vi "test_CCDGetChipTemperature.vi"(8 "error in":errorcluster) -> (0 "error out":errorcluster)   [LabVIEW 2023]
uses:
  <vilib>/addons/_JKI Toolkits/Caraya/classes/Test/Test.lvclass
  <vilib>/addons/_JKI Toolkits/Caraya/classes/Assert/Assert.lvclass
  horiba.test.lvlib
  <vilib>/addons/_JKI Toolkits/Caraya/classes/Assert/Assert Greater_Variant.vi
  <vilib>/addons/_JKI Toolkits/Caraya/classes/Assert/Assert Not Error.vi
  <vilib>/addons/_JKI Toolkits/Caraya/classes/Assert/Assert Less_Variant.vi
  Classes/CCD/CCD.lvclass
  Classes/GenericDevice/GenericDevice.lvclass
panel:
  # "Connector Pane"
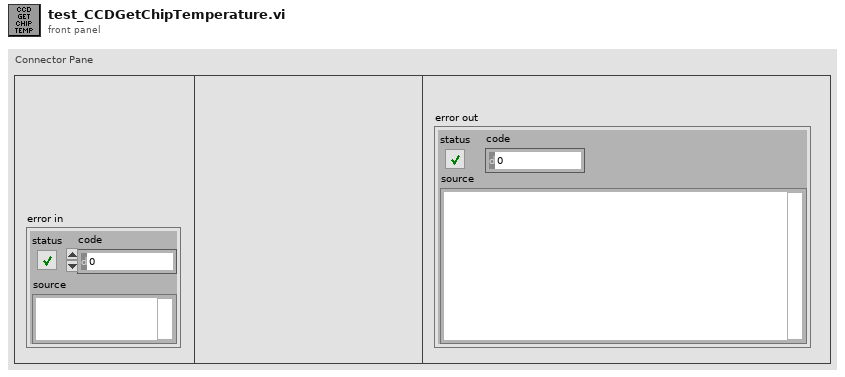
[diagram p1: front panel]
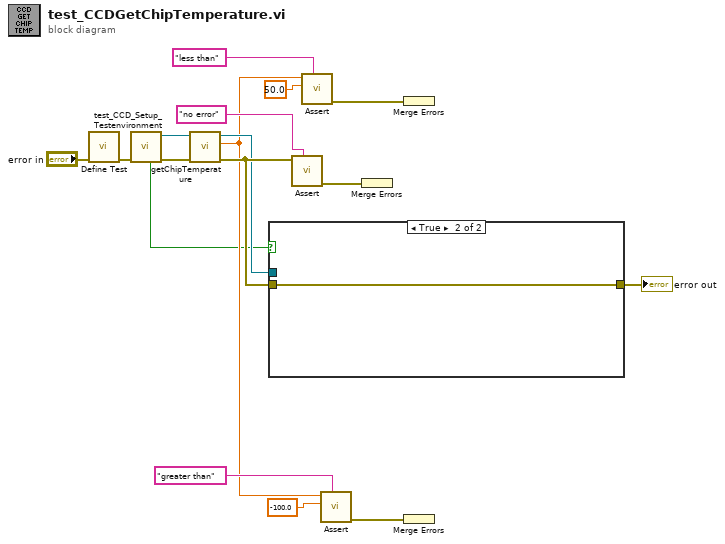
[diagram p0: block diagram]
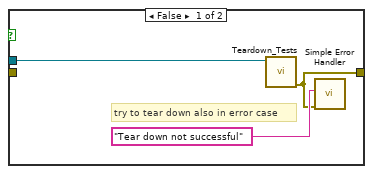
[diagram p2: hidden frame]
diagram:
  n1 = call <vilib>:"Define Test.vi"("error in (no error)"="error in") -> ("error out"=w4:errorcluster)  [unwired: 9 in, 1 out]
  n2 = call "test_CCD_Setup_Testenvironment.vi"("error in"=w4) -> ("error out"=w3:errorcluster, "CCD out"=w2:refnum<class "CCD.lvclass">, "Module Was Already Running?"=w1:bool)  [unwired: 7 in, 1 out]
  n3 = call "getChipTemperature.vi"("error in (no error)"=w3, "CCD in"=w2) -> ("error out"=w10:errorcluster, "temperature °C"=w6:dbl, "CCD out"=w9:refnum<class "CCD.lvclass">)  [unwired: 7 in]
  n4 = case shown="True" w1 {
    tunnel: w9 -> [w19 _]
    tunnel: [w18 w21] -> w5
    tunnel: w10 -> [_ w21]
    frame False {
      # "try to tear down also in error case"
      n5 = call "Teardown_Tests.vi"("horiba.lvlib:GenericDevice"=w19) -> ("error out"=w18:errorcluster)  [unwired: 9 in, 1 out]
      n6 = call <vilib>:"Simple Error Handler.vi"("error source (\" \")"="Tear down not successful" ("error source (\" \")"), "error in (no error)"=w18) -> ()  [unwired: 3 in, 5 out]
    }
    frame True {
    }
  }
  "error out" <- w5
  n7 = call-poly <vilib>:"Assert.vi"("Label"="no error" ("Label (VI Title)"), "Not Error?"=w10) -> ("error out"=w11:errorcluster)  [unwired: 8 in, 1 out]
  n8 = call-poly <vilib>:"Assert.vi"("Label"="less than" ("Label (VI Title)"), "Y"=50.0 ("temperature °C"), "X"=w6) -> ("error out"=w15:errorcluster)  [unwired: 7 in, 1 out]
  n9 = call-poly <vilib>:"Assert.vi"("Label"="greater than" ("Label (VI Title)"), "Y"=-100.0 ("temperature °C"), "X"=w6) -> ("error out"=w16:errorcluster)  [unwired: 7 in, 1 out]
  n10 = Merge Errors(w11) -> ()  [unwired: 1 out]
  n11 = Merge Errors(w15) -> ()  [unwired: 1 out]
  n12 = Merge Errors(w16) -> ()  [unwired: 1 out]
